vi "Teleop Cleaned by Oscar.vi"(10 "Match Info":T5={"Autonomous Elapsed Seconds"=0.0, "TeleOp Elapsed Seconds"=0.0, "Disabled Elapsed Seconds"=0.0, "Visited Autonomous"=FALSE, "Visited TeleOp"=FALSE, "Visited Disabled"=FALSE, "Autonomous Settings"={"Autonomous Style"=enum."Independent", "VI Refnum"=refnum}}, 11 "Call Context":T6) -> ()   [LabVIEW 2017]
doc: "This VI is called for each TeleOp packet received from the DS where the robot is not disabled. It is often used to read from the joysticks and update I/O or to update setpoints for timed control loops. It should complete and return within 20 milliseconds or it may miss DS packets."
uses:
  <vilib>/Rock Robotics/WPI/DriverStation/WPI_DriverStationDerivedRobotMode.ctl
  <vilib>/Rock Robotics/WPI/DriverStation/WPI_DriverStationMatch Info.ctl
  drive enum.ctl
  <vilib>/Rock Robotics/WPI/ThirdParty/Phoenix-LabVIEW/Motor Controller/Controls/CTRE_Phoenix_MotorControl_FeedbackDevice.ctl
  <vilib>/Rock Robotics/WPI/ThirdParty/Phoenix-LabVIEW/Motor Controller/Controls/CTRE_Phoenix_MotorControl_ControlMode.ctl
  <vilib>/Rock Robotics/WPI/Utilities/WPI_GetSetVariantRefNum.vi
  <vilib>/Rock Robotics/Network Tables/NT Write Boolean Array.vi
  <vilib>/Rock Robotics/Network Tables/NT Write Numeric Array.vi
  <vilib>/Rock Robotics/Network Tables/NT Read Boolean.vi
  <vilib>/Rock Robotics/Network Tables/NT Read Number.vi
  <vilib>/Rock Robotics/WPI/ThirdParty/Phoenix-LabVIEW/Motor Controller/Get/CTRE_Phoenix_MotorController_GetOutputCurrent_Enhanced.vi
  <vilib>/Rock Robotics/WPI/ThirdParty/Phoenix-LabVIEW/Motor Controller/Get/CTRE_Phoenix_MotorController_GetVoltage.vi
  <vilib>/Rock Robotics/WPI/ThirdParty/Phoenix-LabVIEW/Motor Controller/Get/CTRE_Phoenix_MotorController_GetClosedLoopData.vi
  <vilib>/Rock Robotics/WPI/ThirdParty/Phoenix-LabVIEW/Motor Controller/Get/CTRE_Phoenix_MotorController_GetSelectedSensorData.vi
panel:
  in  "X and Y values In":bool
  in  "Tab Control":T1(tab)
  in  "Cruise Velocity 3":i32=2000
  in  "Max Acceleration 3":i32=2000
  in  "Cruise Velocity 4":i32=2000
  in  "Max Acceleration 4":i32=2000
  in  "P 3":dbl format="%#_13g"
  in  "I 3":dbl format="%#_13g"
  in  "D 3":dbl format="%#_13g"
  in  "F 3":dbl=0.0095 format="%#_13g"
  in  "P 4":dbl format="%#_13g"
  in  "I 4":dbl format="%#_13g"
  in  "D 4":dbl format="%#_13g"
  in  "F 4":dbl=0.0095 format="%#_13g"
  out "Velocity (Raw Sensor Units per 100 ms) 6":i32
  out "Position (Raw Sensor Units) 6":i32
  out "Percent Output 4":dbl
  out "Velocity (Raw Sensor Units per 100 ms) 5":i32
  out "Position (Raw Sensor Units) 5":i32
  out "Percent Output 3":dbl
  out "Output Current 3":dbl
  out "Closed-loop Error 4":i32
  out "Output Current 4":dbl
  out "Closed-loop Error 3":i32
  in  "P":dbl format="%#_13g"
  in  "I":dbl format="%#_13g"
  in  "D":dbl format="%#_13g"
  in  "F":dbl=0.0095 format="%#_13g"
  in  "Cruise Velocity":i32=2000
  in  "Max Acceleration":i32=2000
  in  "Cruise Velocity 2":i32=2000
  in  "Max Acceleration 2":i32=2000
  in  "P 2":dbl format="%#_13g"
  in  "I 2":dbl format="%#_13g"
  in  "D 2":dbl format="%#_13g"
  in  "F 2":dbl=0.0095 format="%#_13g"
  out "Closed-loop Error 2":i32
  out "Percent Output 2":dbl
  out "Output Current 2":dbl
  out "Velocity (Raw Sensor Units per 100 ms) 4":i32
  out "Position (Raw Sensor Units) 4":i32
  out "Percent Output":dbl
  out "Output Current":dbl
  out "Velocity (Raw Sensor Units per 100 ms) 3":i32
  out "Position (Raw Sensor Units) 3":i32
  out "Closed-loop Error":i32
  out "Velocity (Raw Sensor Units per 100 ms) 7":i32
  out "Position (Raw Sensor Units) 7":i32
  out "Closed-loop Error 5":i32
  out "Percent Output 5":dbl
  out "Output Current 5":dbl
  out "Closed-loop Error 6":i32
  in  "Cruise Velocity 5":i32=2000
  in  "Max Acceleration 5":i32=2000
  in  "Cruise Velocity 6":i32=2000
  in  "Max Acceleration 6":i32=2000
  in  "P 5":dbl format="%#_13g"
  in  "D 5":dbl format="%#_13g"
  in  "F 5":dbl=0.0095 format="%#_13g"
  in  "I 5":dbl format="%#_13g"
  in  "P 6":dbl format="%#_13g"
  in  "I 6":dbl format="%#_13g"
  in  "D 6":dbl format="%#_13g"
  in  "F 6":dbl=0.0095 format="%#_13g"
  out "Velocity (Raw Sensor Units per 100 ms) 8":i32
  out "Position (Raw Sensor Units) 8":i32
  out "Percent Output 6":dbl
  out "Output Current 6":dbl
  out "Position (Raw Sensor Units)":i32
  out "Velocity (Raw Sensor Units per 100 ms)":i32
  out "Position (Raw Sensor Units) 2":i32
  out "Velocity (Raw Sensor Units per 100 ms) 2":i32
  in  "Y axis value":dbl
  in  "X axis value":dbl
  out "encoder position":i32(graph)
  out "X and Y":T2(graph)
  out "horizontal":dbl
  out "joystick output vertical":dbl
  out "closed loop error":T3(graph)
  out "voltage vs current left":T2(graph)
  out "voltage vs current right":T2(graph)
  out "Speed Closed Loop Plots":T4(graph)
  out "Sample Slider 0":dbl(slide) scale=0.0..5.0
  out "Sample Boolean 1":bool
  out "Sample Boolean 0":bool
  # "Joystick"
  # "Front Panel"
  # "what we want"
  # "actual"
  # "0.005740418607"
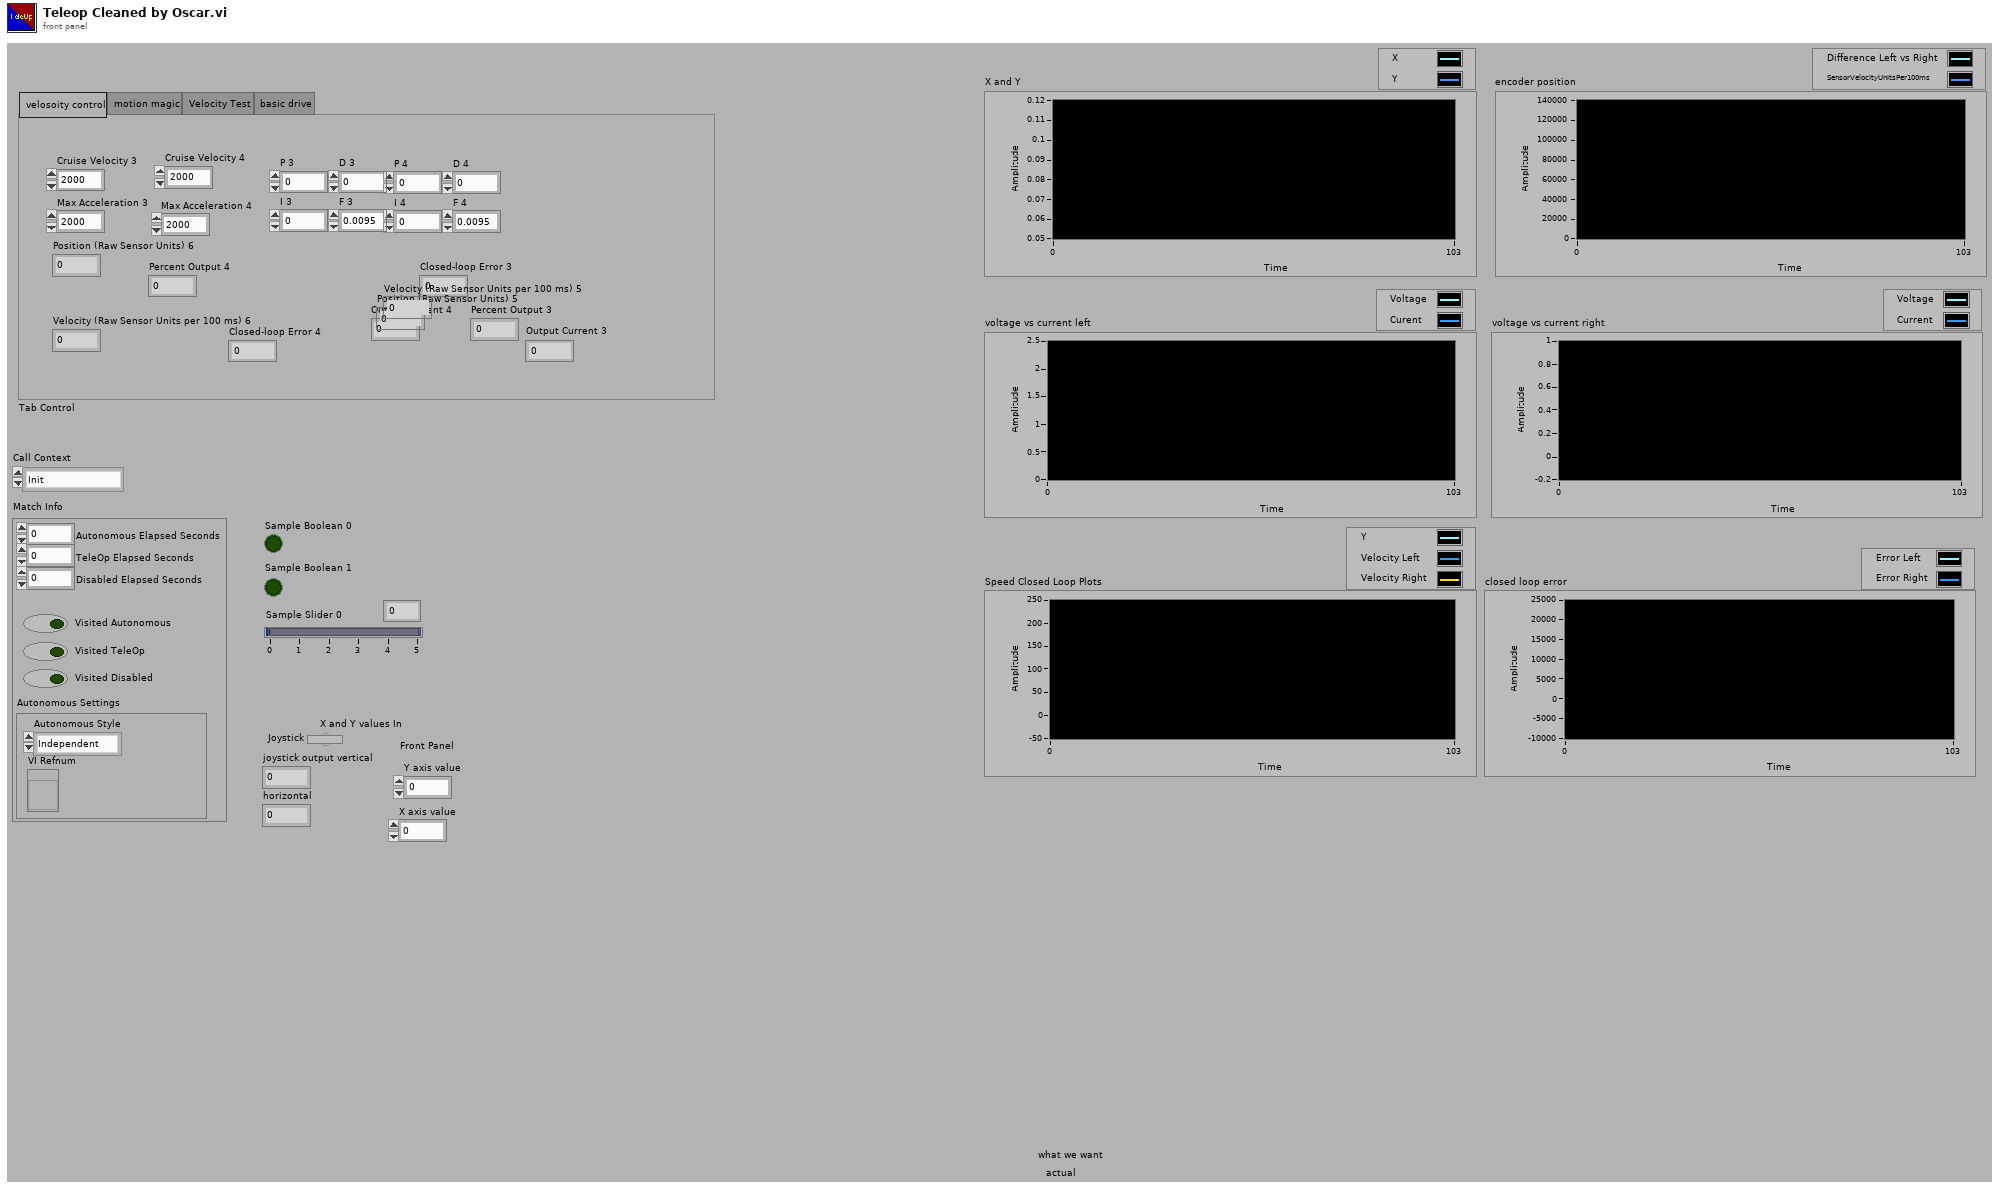
[diagram p1: front panel]
types:
  T1 = enum32{"velosoity control", "motion magic", "Velocity Test", "basic drive"}
  T2 = cluster{"Percent Output":dbl, "Output Current":dbl}
  T3 = cluster{"Closed-loop Error":i32, "Closed-loop Error":i32}
  T4 = cluster{dbl, "Velocity (Raw Sensor Units per 100 ms)":i32, "Velocity (Raw Sensor Units per 100 ms)":i32}
  T5 = typedef "WPI_DriverStationMatch Info.ctl" = cluster{"Autonomous Elapsed Seconds":dbl, "TeleOp Elapsed Seconds":dbl, "Disabled Elapsed Seconds":dbl, "Visited Autonomous":bool, "Visited TeleOp":bool, "Visited Disabled":bool, "Autonomous Settings":cluster{"Autonomous Style":enum16{"Iterative", "Independent"}, "VI Refnum":refnum<vi>}}
  T6 = typedef "WPI_DriverStationDerivedRobotMode.ctl" = enum16{"Init", "Execute", "Stop"}
  T7 = typedef "drive enum.ctl" = enum16{"velosoity control", "motion magic", "Velocity Test", "basic drive"}
  T8 = typedef "WPI_JoystickDevRef.ctl" = cluster{"Device":T9}
  T9 = typedef "WPI_JoystickDeviceEnum.ctl" = enum16{"USB 0", "USB 1", "USB 2", "USB 3", "USB 4", "USB 5"}
  T10 = typedef "WPI_RobotDriveDevRef.ctl" = cluster{"DevStatus":errorcluster, "Motors[]":T11[], "Square Inputs":bool, "Max Output":dbl}
  T11 = typedef "WPI_MotorControlDeviceRef.ctl" = cluster{"DeviceStatus":errorcluster, "Type":T12, "PWM":cluster{"PWM Channel":T13, "DeadBand":T14}, "CAN":cluster{"Device Number":u8, "SetOutput VI Ref":variant, "GetOutput VI Ref":variant, "Enable VI Ref":variant, "Disable VI Ref":variant, "Data":variant}, "Invert":bool, "DIO PWM":cluster{"PWM \"Enable\" Channel":T13, "DIOChannel":T15, "PWM Rate":dbl}}
  T12 = typedef "WPI_MotorControlType.ctl" = enum16{"PWM", "CAN", "DIO PWM"}
  T13 = typedef "FPGA_DIOPWMChannel.ctl" = enum8{"PWM 0", "PWM 1", "PWM 2", "PWM 3", "PWM 4", "PWM 5", "PWM 6", "PWM 7", "PWM 8", "PWM 9", "PWM MXP 0", "PWM MXP 1", "PWM MXP 2", "PWM MXP 3", "PWM MXP 4", "PWM MXP 5", "PWM MXP 6", "PWM MXP 7", "PWM MXP 8", "PWM MXP 9", "Invalid"}
  T14 = typedef "WPI_PWMDeadband.ctl" = cluster{"Name":string, "maxPositivePwm":i32, "minPositivePwm":i32, "centerPwm":i32, "maxNegativePwm":i32, "minNegativePwm":i32, "angularRange":u16}
  T15 = typedef "FPGA_DIOChannel.ctl" = enum8{"DIO 0", "DIO 1", "DIO 2", "DIO 3", "DIO 4", "DIO 5", "DIO 6", "DIO 7", "DIO 8", "DIO 9", "DIO MXP 0", "DIO MXP 1", "DIO MXP 2", "DIO MXP 3", "DIO MXP 4", "DIO MXP 5", "DIO MXP 6", "DIO MXP 7", "DIO MXP 8", "DIO MXP 9", "DIO MXP 10", "DIO MXP 11", "DIO MXP 12", "DIO MXP 13", "DIO MXP 14", "DIO MXP 15", "SPI Port CS1", "SPI Port CS2", "SPI Port CS3", "SPI Port MISO", "SPI Port MOSI", "Invalid"}
  T16 = typedef "CTRE_Phoenix_MotorControl_ControlMode.ctl" = u16
  T17 = typedef "CTRE_Phoenix_MotorControl_FeedbackDevice.ctl" = i8
  T18 = cluster{"Y axis value":dbl, "Velocity (Raw Sensor Units per 100 ms)":i32, "Velocity (Raw Sensor Units per 100 ms)":i32}
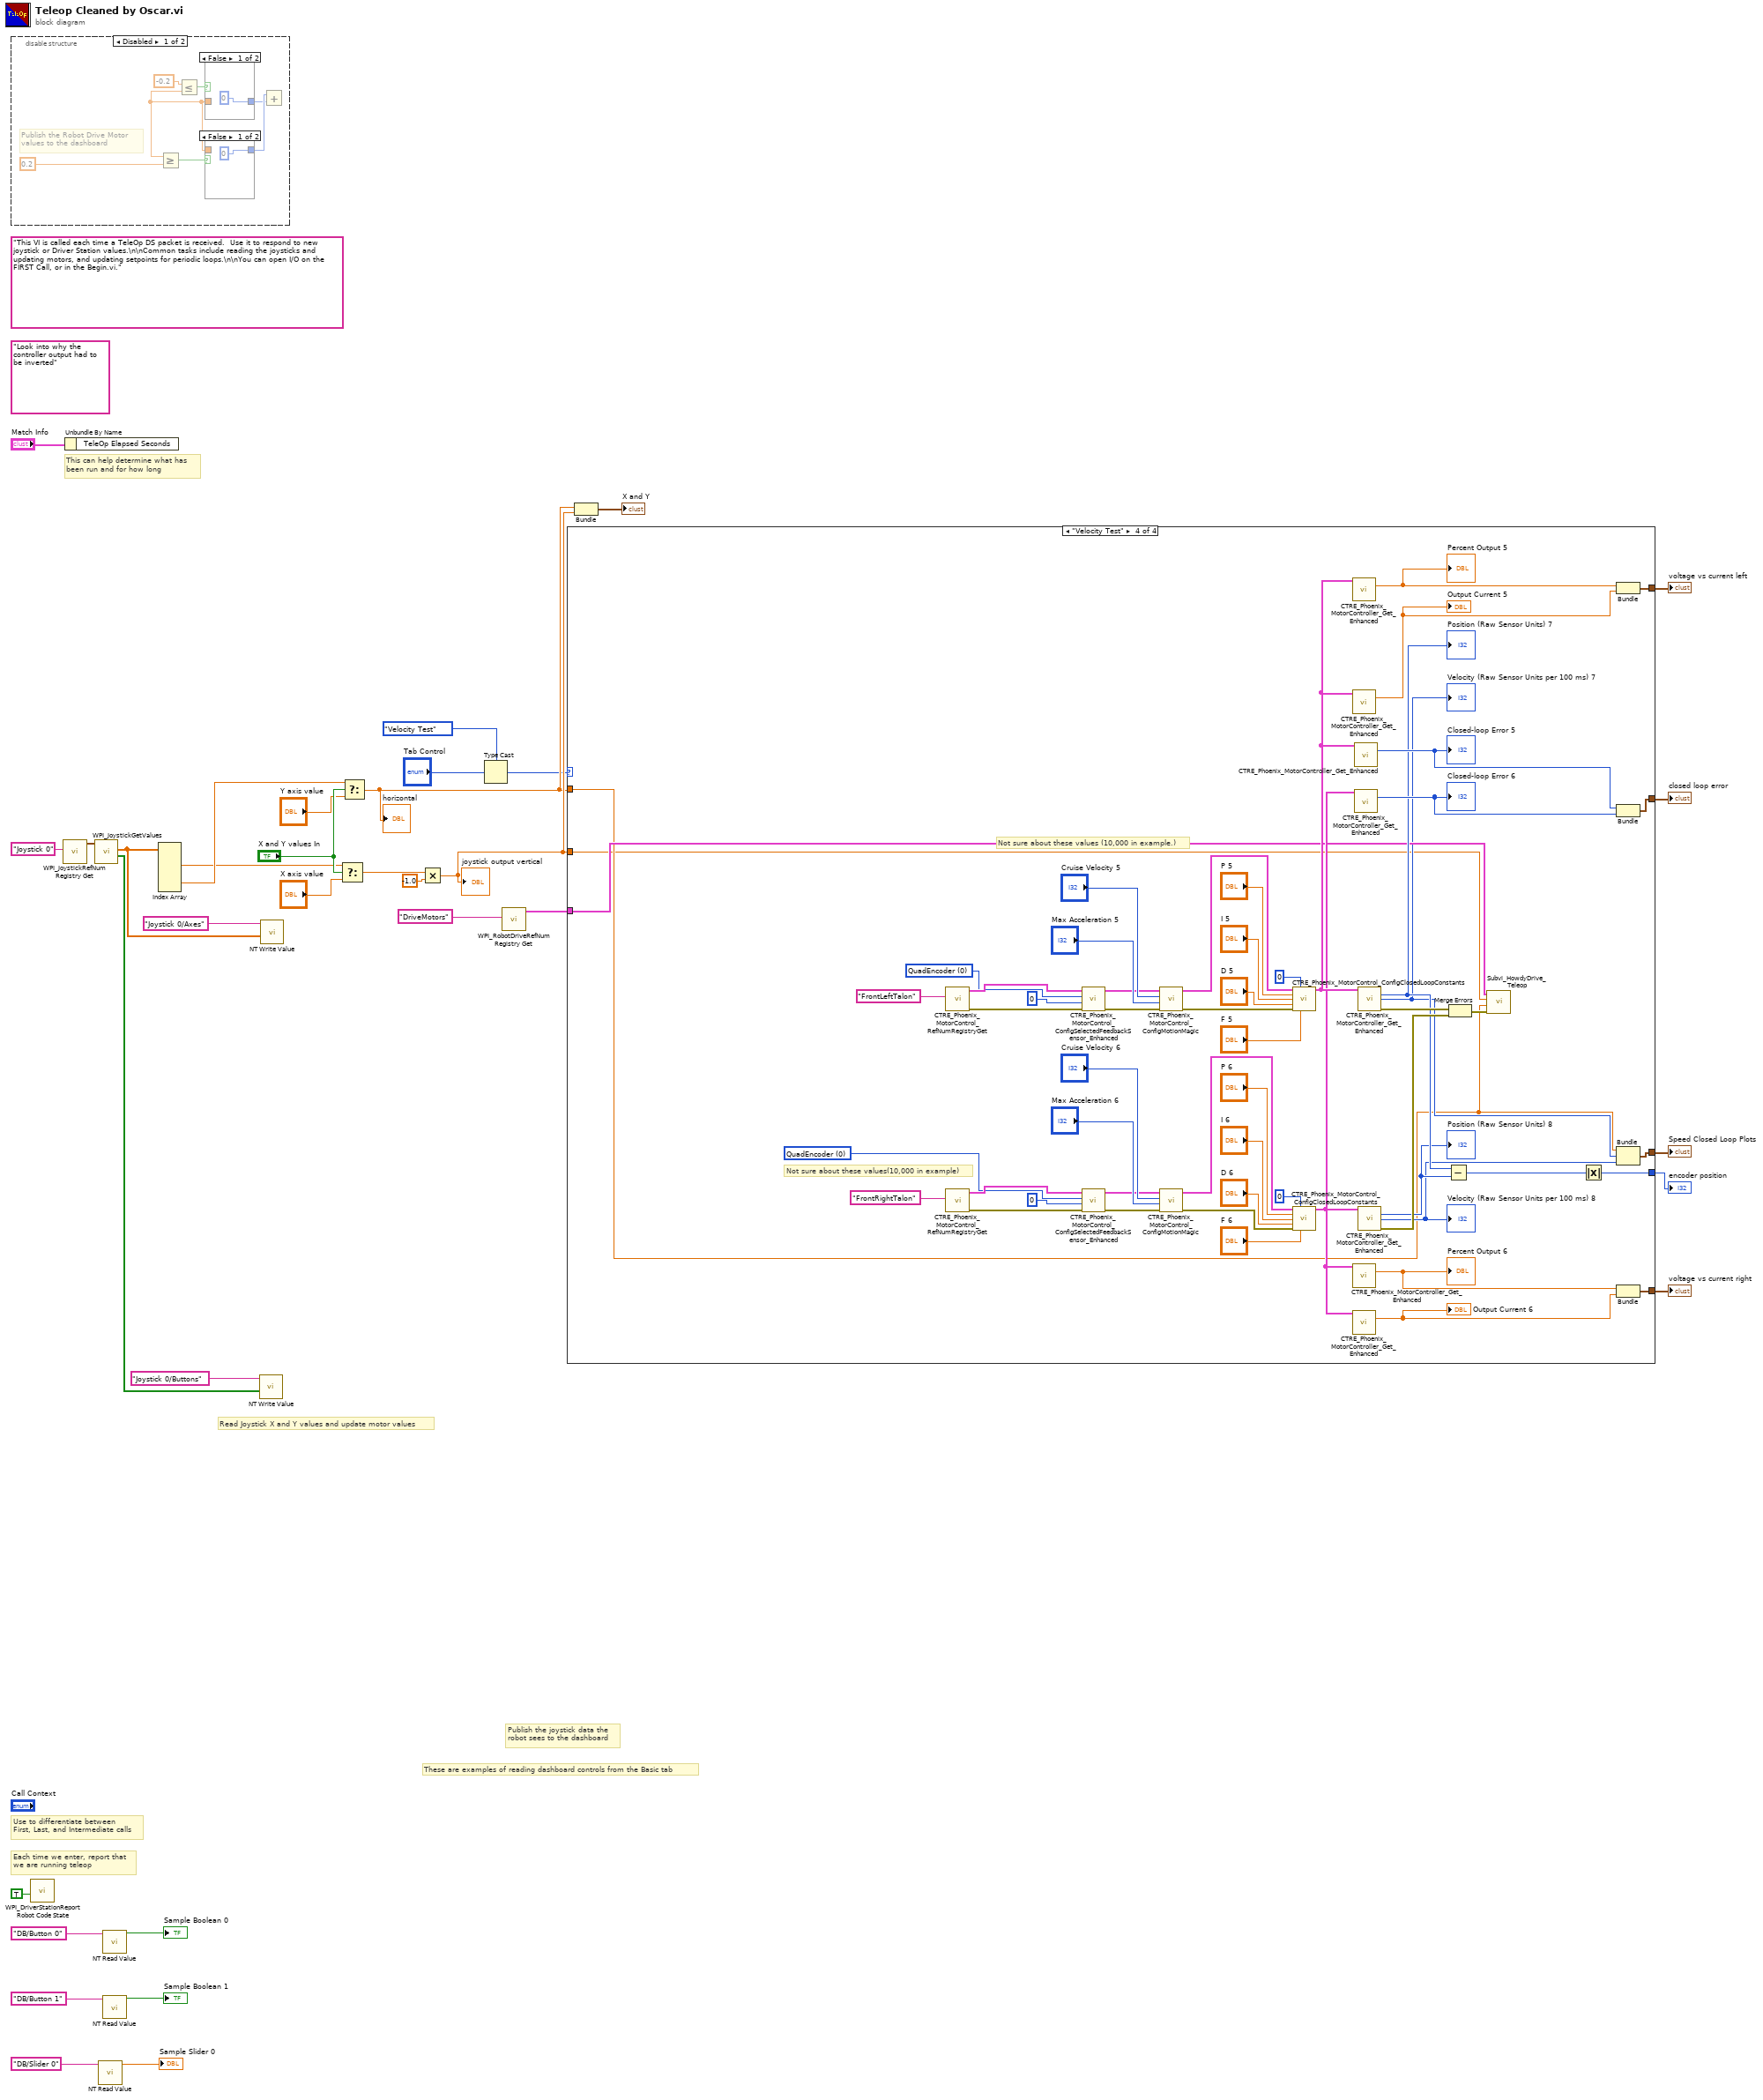
[diagram p0: block diagram]
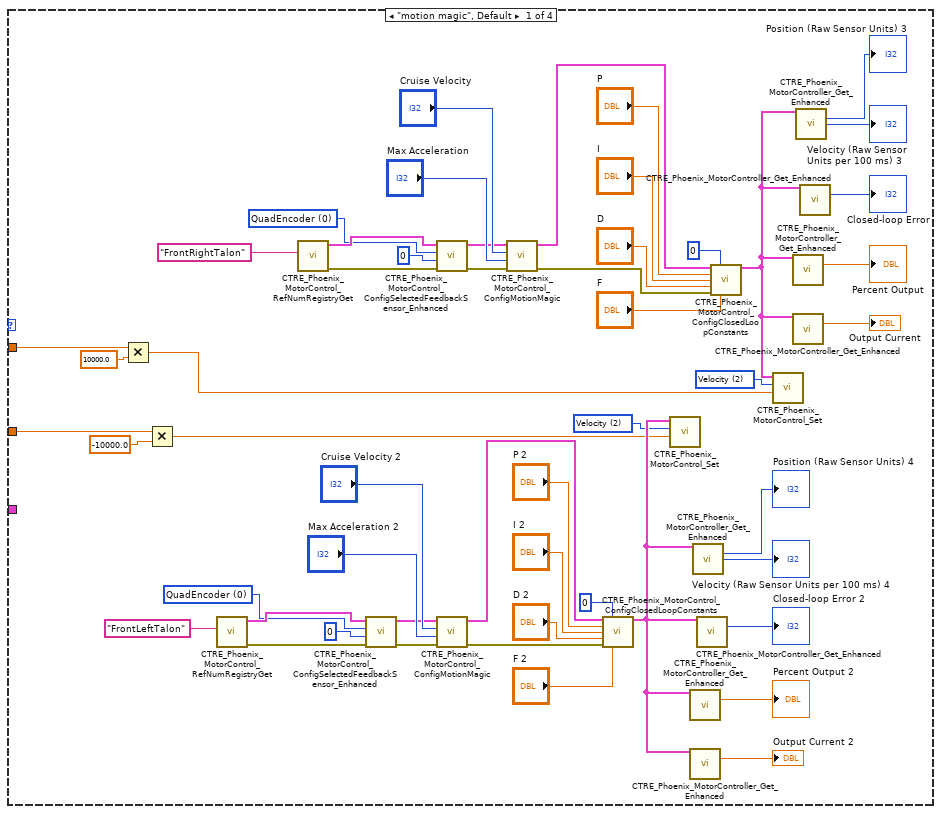
[diagram p5: hidden frame]
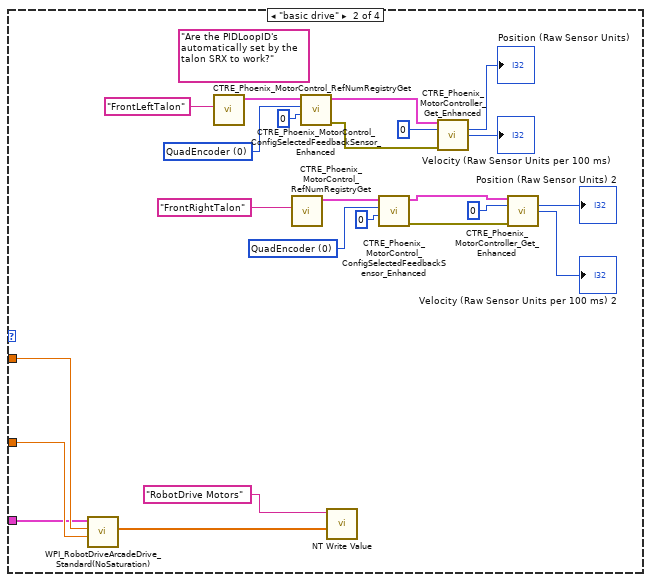
[diagram p6: hidden frame]
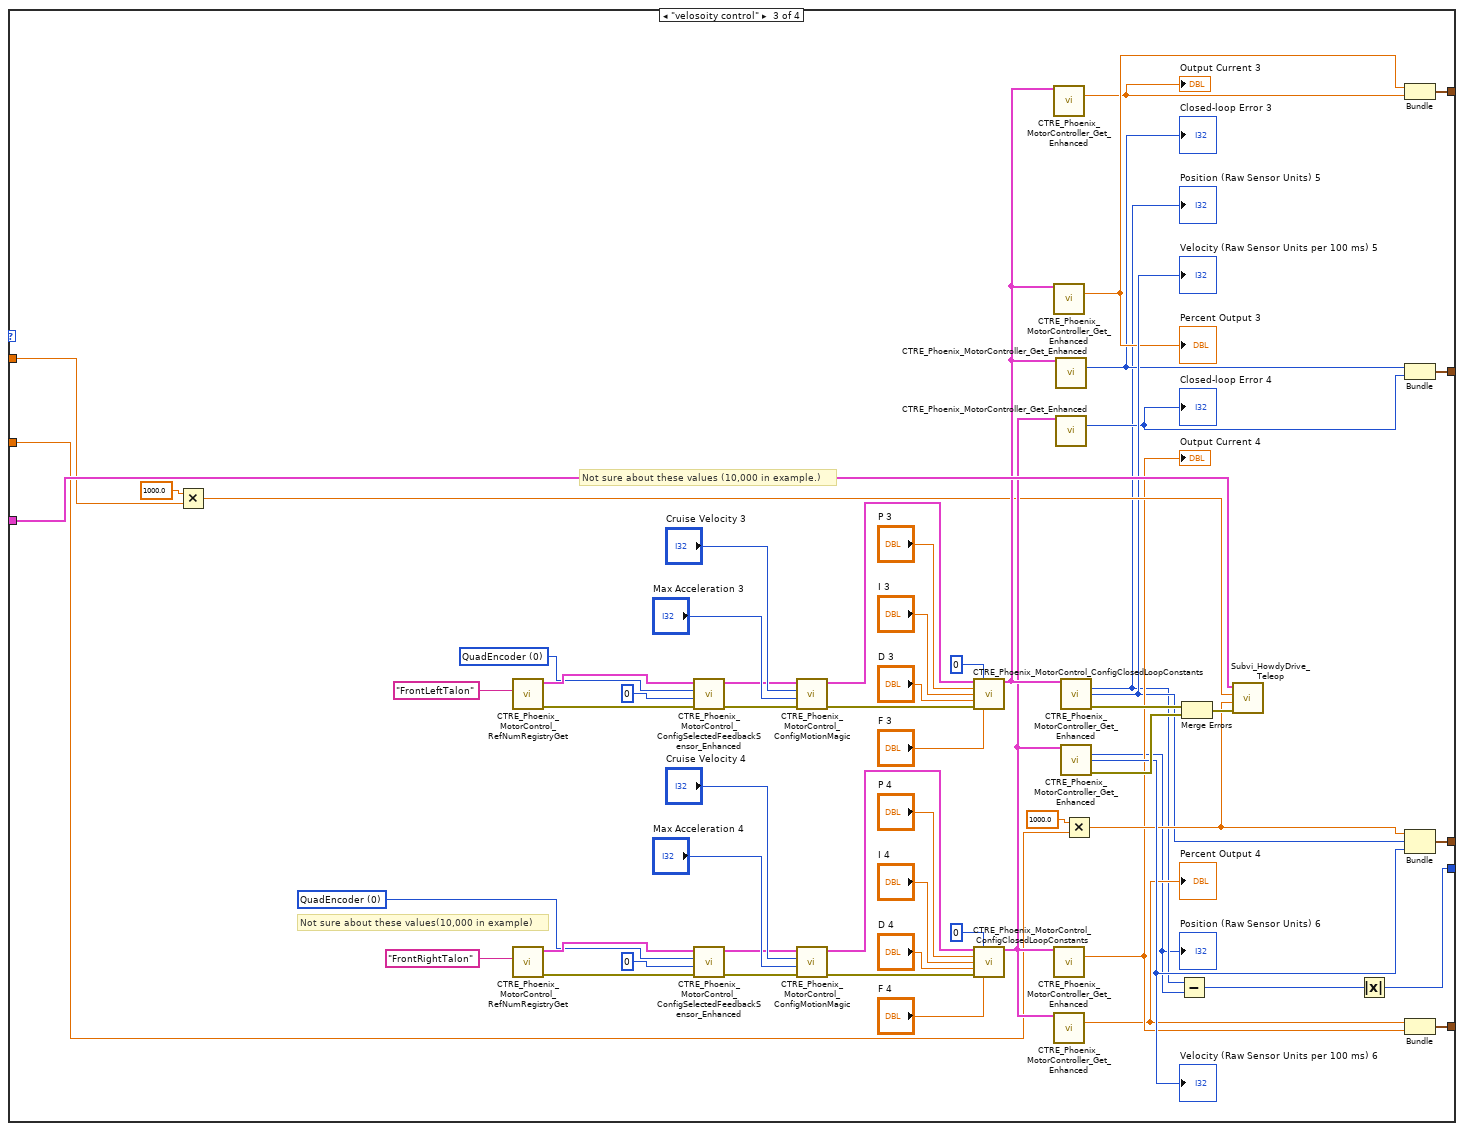
[diagram p7: hidden frame]
diagram:
  (unwired) "Look into why the controller output had to be inverted"
  (unwired) "This VI is called each time a TeleOp DS packet is received.  Use it to respond to new joystick or Driver Station values.\n\nCommon tasks include reading the joysticks and updating motors, and updating setpoints for periodic loops.\n\nYou can open I/O on the FIRST Call, or in the Begin.vi."
  # "These are examples of reading dashboard controls from the Basic tab"
  # "Publish the joystick data the\nrobot sees to the dashboard"
  # "Read Joystick X and Y values and update motor values"
  # "Each time we enter, report that\nwe are running teleop"
  # "Use to differentiate between\nFirst, Last, and Intermediate calls"
  # "This can help determine what has\nbeen run and for how long"
  n1 = disable-structure shown="Disabled" {
    frame Disabled {
      # "Publish the Robot Drive Motor\nvalues to the dashboard"
      n2 = Greater Or Equal?(y=0.2) -> (x=w37:dbl, x >= y?=w40:bool)
      n3 = Less Or Equal?(x=-0.2, y=w37) -> (x <= y?=w38:bool)
      n4 = case shown="False" w38 {
        tunnel: w37 -> [_ w43]
        tunnel: [0 w43] -> w35
        frame False {
        }
        frame True {
        }
      }
      n5 = case shown="False" w40 {
        tunnel: [0 w45] -> w36
        tunnel: w37 -> [_ w45]
        frame False {
        }
        frame True {
        }
      }
      n6 = Add(x=w36, y=w35) -> ()  [unwired: 1 out]
    }
    frame Enabled {
    }
  }
  n7 = call <vilib>:"WPI_DriverStationReport Robot Code State.vi"("TeleOp"=TRUE ("Autonomous")) -> ()  [unwired: 10 in, 1 out]
  n8 = call <vilib>:"WPI_JoystickRefNum Registry Get.vi"("refnum name"="Joystick 0") -> ("JoystickDevRef"=w30:T8)  [unwired: 1 in, 9 out]
  n9 = Unbundle By Name("Match Info") -> ()  [unwired: 1 out]
  n10 = call <vilib>:"WPI_JoystickGetValues.vi"("JoystickDevRef"=w30) -> ("Buttons"=w26:bool[], "Axes"=w27:dbl[])  [unwired: 6 in, 3 out]
  n11 = call-poly <vilib>:"NT Read Value.vi"("Name"="DB/Slider 0" ("refnum name")) -> ("Numeric"=→"Sample Slider 0":dbl)  [unwired: 9 in, 1 out]
  n12 = call-poly <vilib>:"NT Read Value.vi"("Name"="DB/Button 0" ("refnum name")) -> ("Boolean"=→"Sample Boolean 0":bool)  [unwired: 9 in, 1 out]
  n13 = call-poly <vilib>:"NT Read Value.vi"("Name"="DB/Button 1" ("refnum name")) -> ("Boolean"=→"Sample Boolean 1":bool)  [unwired: 9 in, 1 out]
  n14 = Index Array(array=w27) -> (element #2=w7:dbl, element #5=w8:dbl)  [unwired: 6 in, 4 out]
  n15 = call-poly <vilib>:"NT Write Value.vi"("Boolean Array"=w26, "Name"="Joystick 0/Buttons") -> ()  [unwired: 9 in, 1 out]
  n16 = call-poly <vilib>:"NT Write Value.vi"("Numeric Array"=w27, "Name"="Joystick 0/Axes") -> ()  [unwired: 9 in, 1 out]
  n17 = Select(t=w7, s="X and Y values In", f="X axis value") -> (s? t:f=w4:dbl)
  n18 = Select(t=w8, s="X and Y values In", f="Y axis value") -> (s? t:f=w5:dbl)
  "horizontal" <- w5
  n19 = Multiply(x=w4, y=-1.0) -> (x*y=w16:dbl)
  "joystick output vertical" <- w16
  n20 = Type Cast(type=drive_enum."Velocity Test", x="Tab Control") -> (*(type *) &x=w1:T7)
  n21 = call <vilib>:"WPI_RobotDriveRefNum Registry Get.vi"("refnum name"="DriveMotors") -> ("RobotDriveDevRef"=w18:T10)  [unwired: 1 in, 9 out]
  n22 = case shown="\"Velocity Test\"" w1 {
    tunnel: w16 -> [w48 w101 w139 w181]
    tunnel: w5 -> [w51 w100 w140 w182]
    tunnel: w18 -> [_ w99 w180 w190]
    tunnel: [_ _ w125 w189] -> w15
    tunnel: [_ _ w123 w187] -> w14
    tunnel: [_ _ w122 w185] -> w13
    tunnel: [_ _ w121 w186] -> w12
    tunnel: [_ _ w124 w188] -> w11
    frame "motion magic", Default {
      w56 = T16 2 items=["PercentOutput"=0, "Position"=1, "Velocity"=2, "Current"=3, "Follower"=5, "MotionProfile"=6, "MotionMagic"=7, "MotionMagicArc"=8, "MotionProfileArc"=10, "Disabled"=15] ("Control Mode")
      w53 = T17 0 items=["None"=-1, "QuadEncoder"=0, "Analog"=2, "Tachometer"=4, "Pulse Width Encoded Position"=8, "Sensor Sum (S0 + S1)"=9, "Sensor Difference (D0 - D1)"=10, "Remote Source 0"=11, "Remote Source 1"=12, "Software Emulated"=15] ("Feedback Device")
      w79 = T16 2 items=["PercentOutput"=0, "Position"=1, "Velocity"=2, "Current"=3, "Follower"=5, "MotionProfile"=6, "MotionMagic"=7, "MotionMagicArc"=8, "MotionProfileArc"=10, "Disabled"=15] ("Control Mode")
      w76 = T17 0 items=["None"=-1, "QuadEncoder"=0, "Analog"=2, "Tachometer"=4, "Pulse Width Encoded Position"=8, "Sensor Sum (S0 + S1)"=9, "Sensor Difference (D0 - D1)"=10, "Remote Source 0"=11, "Remote Source 1"=12, "Software Emulated"=15] ("Feedback Device")
      n23 = Multiply(x=w51, y=10000.0) -> (x*y=w46:dbl)
      n24 = Multiply(x=w48, y=-10000.0) -> (x*y=w47:dbl)
      n25 = call <vilib>:"CTRE_Phoenix_MotorControl_RefNumRegistryGet.vi"("refnum name"="FrontLeftTalon") -> ("error out"=w81:errorcluster, "PhoenixMotorControlDevRef"=w80:T11)  [unwired: 9 in]
      n26 = call <vilib>:"CTRE_Phoenix_MotorControl_RefNumRegistryGet.vi"("refnum name"="FrontRightTalon") -> ("error out"=w58:errorcluster, "PhoenixMotorControlDevRef"=w57:T11)  [unwired: 9 in]
      n27 = call <vilib>:"CTRE_Phoenix_MotorControl_ConfigSelectedFeedbackSensor_Enhanced.vi"("error in (no error)"=w81, "pidLoopIdx"=0, "Feedback Device"=w76, "PhoenixMotorControlDevRef"=w80) -> ("error out"=w83:errorcluster, "PhoenixMotorControlDevRef"=w82:T11)  [unwired: 6 in]
      n28 = call <vilib>:"CTRE_Phoenix_MotorControl_ConfigSelectedFeedbackSensor_Enhanced.vi"("error in (no error)"=w58, "pidLoopIdx"=0, "Feedback Device"=w53, "PhoenixMotorControlDevRef"=w57) -> ("error out"=w60:errorcluster, "PhoenixMotorControlDevRef"=w59:T11)  [unwired: 6 in]
      n29 = call <vilib>:"CTRE_Phoenix_MotorControl_ConfigMotionMagic.vi"("error in (no error)"=w83, "Acceleration"="Max Acceleration 2", "Cruise Velocity"="Cruise Velocity 2", "PhoenixMotorControlDevRef"=w82) -> ("error out"=w94:errorcluster, "PhoenixMotorControlDevRef"=w93:T11)  [unwired: 6 in]
      n30 = call <vilib>:"CTRE_Phoenix_MotorControl_ConfigMotionMagic.vi"("error in (no error)"=w60, "Acceleration"="Max Acceleration", "Cruise Velocity"="Cruise Velocity", "PhoenixMotorControlDevRef"=w59) -> ("error out"=w62:errorcluster, "PhoenixMotorControlDevRef"=w61:T11)  [unwired: 6 in]
      n31 = call <vilib>:"CTRE_Phoenix_MotorControl_ConfigClosedLoopConstants.vi"("PhoenixMotorControlDevRef"=w93, "slotIdx"=0, "P"="P 2", "I"="I 2", "D"="D 2", "error in (no error)"=w94, "F"="F 2") -> ("PhoenixMotorControlDevRef"=w97:T11)  [unwired: 7 in, 1 out]
      n32 = call <vilib>:"CTRE_Phoenix_MotorControl_Set.vi"("Output"=w47, "Control Mode"=w79, "PhoenixMotorControlDevRef"=w97) -> ()  [unwired: 7 in, 2 out]
      n33 = call-poly <vilib>:"CTRE_Phoenix_MotorController_Get_Enhanced.vi"("PhoenixMotorControlDevRef"=w97) -> ("Percent Output"=→"Percent Output 2":dbl)  [unwired: 10 in, 4 out]
      n34 = call-poly <vilib>:"CTRE_Phoenix_MotorController_Get_Enhanced.vi"("PhoenixMotorControlDevRef"=w97) -> ("Output Current"=→"Output Current 2":dbl)  [unwired: 12 in, 2 out]
      n35 = call-poly <vilib>:"CTRE_Phoenix_MotorController_Get_Enhanced.vi"("PhoenixMotorControlDevRef"=w97) -> ("Position (Raw Sensor Units)"=→"Position (Raw Sensor Units) 4":i32, "Velocity (Raw Sensor Units per 100 ms)"=→"Velocity (Raw Sensor Units per 100 ms) 4":i32)  [unwired: 11 in, 2 out]
      n36 = call-poly <vilib>:"CTRE_Phoenix_MotorController_Get_Enhanced.vi"("PhoenixMotorControlDevRef"=w97) -> ("Closed-loop Error"=→"Closed-loop Error 2":i32)  [unwired: 9 in, 5 out]
      n37 = call <vilib>:"CTRE_Phoenix_MotorControl_ConfigClosedLoopConstants.vi"("PhoenixMotorControlDevRef"=w61, "slotIdx"=0, "P"="P", "I"="I", "D"="D", "error in (no error)"=w62, "F"="F") -> ("PhoenixMotorControlDevRef"=w74:T11)  [unwired: 7 in, 1 out]
      n38 = call <vilib>:"CTRE_Phoenix_MotorControl_Set.vi"("Output"=w46, "Control Mode"=w56, "PhoenixMotorControlDevRef"=w74) -> ()  [unwired: 7 in, 2 out]
      n39 = call-poly <vilib>:"CTRE_Phoenix_MotorController_Get_Enhanced.vi"("PhoenixMotorControlDevRef"=w74) -> ("Percent Output"=→"Percent Output":dbl)  [unwired: 10 in, 4 out]
      n40 = call-poly <vilib>:"CTRE_Phoenix_MotorController_Get_Enhanced.vi"("PhoenixMotorControlDevRef"=w74) -> ("Output Current"=→"Output Current":dbl)  [unwired: 12 in, 2 out]
      n41 = call-poly <vilib>:"CTRE_Phoenix_MotorController_Get_Enhanced.vi"("PhoenixMotorControlDevRef"=w74) -> ("Position (Raw Sensor Units)"=→"Position (Raw Sensor Units) 3":i32, "Velocity (Raw Sensor Units per 100 ms)"=→"Velocity (Raw Sensor Units per 100 ms) 3":i32)  [unwired: 11 in, 2 out]
      n42 = call-poly <vilib>:"CTRE_Phoenix_MotorController_Get_Enhanced.vi"("PhoenixMotorControlDevRef"=w74) -> ("Closed-loop Error"=→"Closed-loop Error":i32)  [unwired: 9 in, 5 out]
    }
    frame "basic drive" {
      (unwired) "Are the PIDLoopID's automatically set by the talon SRX to work?"
      w113 = T17 0 items=["None"=-1, "QuadEncoder"=0, "Analog"=2, "Tachometer"=4, "Pulse Width Encoded Position"=8, "Sensor Sum (S0 + S1)"=9, "Sensor Difference (D0 - D1)"=10, "Remote Source 0"=11, "Remote Source 1"=12, "Software Emulated"=15] ("Feedback Device")
      w120 = T17 0 items=["None"=-1, "QuadEncoder"=0, "Analog"=2, "Tachometer"=4, "Pulse Width Encoded Position"=8, "Sensor Sum (S0 + S1)"=9, "Sensor Difference (D0 - D1)"=10, "Remote Source 0"=11, "Remote Source 1"=12, "Software Emulated"=15] ("Feedback Device")
      n43 = call <vilib>:"WPI_RobotDriveArcadeDrive_Standard(NoSaturation).vi"("Y axis value"=w101, "X axis value"=w100, "RobotDriveDevRef"=w99) -> ("Motor Values"=w102:dbl[])  [unwired: 1 in, 7 out]
      n44 = call <vilib>:"CTRE_Phoenix_MotorControl_RefNumRegistryGet.vi"("refnum name"="FrontLeftTalon") -> ("PhoenixMotorControlDevRef"=w114:T11)  [unwired: 9 in, 1 out]
      n45 = call <vilib>:"CTRE_Phoenix_MotorControl_RefNumRegistryGet.vi"("refnum name"="FrontRightTalon") -> ("PhoenixMotorControlDevRef"=w106:T11)  [unwired: 9 in, 1 out]
      n46 = call <vilib>:"CTRE_Phoenix_MotorControl_ConfigSelectedFeedbackSensor_Enhanced.vi"("pidLoopIdx"=0, "Feedback Device"=w120, "PhoenixMotorControlDevRef"=w114) -> ("error out"=w118:errorcluster, "PhoenixMotorControlDevRef"=w119:T11)  [unwired: 7 in]
      n47 = call-poly <vilib>:"NT Write Value.vi"("Numeric Array"=w102, "Name"="RobotDrive Motors") -> ()  [unwired: 9 in, 1 out]
      n48 = call <vilib>:"CTRE_Phoenix_MotorControl_ConfigSelectedFeedbackSensor_Enhanced.vi"("pidLoopIdx"=0, "Feedback Device"=w113, "PhoenixMotorControlDevRef"=w106) -> ("error out"=w111:errorcluster, "PhoenixMotorControlDevRef"=w112:T11)  [unwired: 7 in]
      n49 = call-poly <vilib>:"CTRE_Phoenix_MotorController_Get_Enhanced.vi"("PhoenixMotorControlDevRef"=w119, "pidLoopIdx"=u32 0, "error in"=w118) -> ("Position (Raw Sensor Units)"=→"Position (Raw Sensor Units)":i32, "Velocity (Raw Sensor Units per 100 ms)"=→"Velocity (Raw Sensor Units per 100 ms)":i32)  [unwired: 9 in, 2 out]
      n50 = call-poly <vilib>:"CTRE_Phoenix_MotorController_Get_Enhanced.vi"("PhoenixMotorControlDevRef"=w112, "pidLoopIdx"=u32 0, "error in"=w111) -> ("Position (Raw Sensor Units)"=→"Position (Raw Sensor Units) 2":i32, "Velocity (Raw Sensor Units per 100 ms)"=→"Velocity (Raw Sensor Units per 100 ms) 2":i32)  [unwired: 9 in, 2 out]
    }
    frame "velosoity control" {
      w147 = T17 0 items=["None"=-1, "QuadEncoder"=0, "Analog"=2, "Tachometer"=4, "Pulse Width Encoded Position"=8, "Sensor Sum (S0 + S1)"=9, "Sensor Difference (D0 - D1)"=10, "Remote Source 0"=11, "Remote Source 1"=12, "Software Emulated"=15] ("Feedback Device")
      w164 = T17 0 items=["None"=-1, "QuadEncoder"=0, "Analog"=2, "Tachometer"=4, "Pulse Width Encoded Position"=8, "Sensor Sum (S0 + S1)"=9, "Sensor Difference (D0 - D1)"=10, "Remote Source 0"=11, "Remote Source 1"=12, "Software Emulated"=15] ("Feedback Device")
      # "Not sure about these values (10,000 in example.)"
      # "Not sure about these values(10,000 in example)"
      n51 = Multiply(x=1000.0, y=w140) -> (x*y=w138:dbl)
      n52 = call <vilib>:"CTRE_Phoenix_MotorControl_RefNumRegistryGet.vi"("refnum name"="FrontLeftTalon") -> ("error out"=w168:errorcluster, "PhoenixMotorControlDevRef"=w167:T11)  [unwired: 9 in]
      n53 = call <vilib>:"CTRE_Phoenix_MotorControl_RefNumRegistryGet.vi"("refnum name"="FrontRightTalon") -> ("error out"=w151:errorcluster, "PhoenixMotorControlDevRef"=w150:T11)  [unwired: 9 in]
      n54 = call <vilib>:"CTRE_Phoenix_MotorControl_ConfigSelectedFeedbackSensor_Enhanced.vi"("error in (no error)"=w168, "pidLoopIdx"=0, "Feedback Device"=w164, "PhoenixMotorControlDevRef"=w167) -> ("error out"=w170:errorcluster, "PhoenixMotorControlDevRef"=w169:T11)  [unwired: 6 in]
      n55 = call <vilib>:"CTRE_Phoenix_MotorControl_ConfigSelectedFeedbackSensor_Enhanced.vi"("error in (no error)"=w151, "pidLoopIdx"=0, "Feedback Device"=w147, "PhoenixMotorControlDevRef"=w150) -> ("error out"=w153:errorcluster, "PhoenixMotorControlDevRef"=w152:T11)  [unwired: 6 in]
      n56 = call <vilib>:"CTRE_Phoenix_MotorControl_ConfigMotionMagic.vi"("error in (no error)"=w170, "Acceleration"="Max Acceleration 3", "Cruise Velocity"="Cruise Velocity 3", "PhoenixMotorControlDevRef"=w169) -> ("error out"=w176:errorcluster, "PhoenixMotorControlDevRef"=w175:T11)  [unwired: 6 in]
      n57 = call <vilib>:"CTRE_Phoenix_MotorControl_ConfigMotionMagic.vi"("error in (no error)"=w153, "Acceleration"="Max Acceleration 4", "Cruise Velocity"="Cruise Velocity 4", "PhoenixMotorControlDevRef"=w152) -> ("error out"=w155:errorcluster, "PhoenixMotorControlDevRef"=w154:T11)  [unwired: 6 in]
      n58 = call <vilib>:"CTRE_Phoenix_MotorControl_ConfigClosedLoopConstants.vi"("PhoenixMotorControlDevRef"=w175, "slotIdx"=0, "P"="P 3", "I"="I 3", "D"="D 3", "error in (no error)"=w176, "F"="F 3") -> ("PhoenixMotorControlDevRef"=w179:T11)  [unwired: 7 in, 1 out]
      n59 = call <vilib>:"CTRE_Phoenix_MotorControl_ConfigClosedLoopConstants.vi"("PhoenixMotorControlDevRef"=w154, "slotIdx"=0, "P"="P 4", "I"="I 4", "D"="D 4", "error in (no error)"=w155, "F"="F 4") -> ("PhoenixMotorControlDevRef"=w162:T11)  [unwired: 7 in, 1 out]
      n60 = call-poly <vilib>:"CTRE_Phoenix_MotorController_Get_Enhanced.vi"("PhoenixMotorControlDevRef"=w179) -> ("Output Current"=w131:dbl)  [unwired: 12 in, 2 out]
      "Output Current 3" <- w131
      n61 = call-poly <vilib>:"CTRE_Phoenix_MotorController_Get_Enhanced.vi"("PhoenixMotorControlDevRef"=w179) -> ("Percent Output"=w132:dbl)  [unwired: 10 in, 4 out]
      "Percent Output 3" <- w132
      n62 = call-poly <vilib>:"CTRE_Phoenix_MotorController_Get_Enhanced.vi"("PhoenixMotorControlDevRef"=w162) -> ("Output Current"=w135:dbl)  [unwired: 12 in, 2 out]
      "Output Current 4" <- w135
      n63 = call-poly <vilib>:"CTRE_Phoenix_MotorController_Get_Enhanced.vi"("PhoenixMotorControlDevRef"=w162) -> ("Percent Output"=w134:dbl)  [unwired: 10 in, 4 out]
      "Percent Output 4" <- w134
      n64 = call-poly <vilib>:"CTRE_Phoenix_MotorController_Get_Enhanced.vi"("PhoenixMotorControlDevRef"=w179) -> ("Closed-loop Error"=w130:i32)  [unwired: 9 in, 5 out]
      "Closed-loop Error 3" <- w130
      n65 = call-poly <vilib>:"CTRE_Phoenix_MotorController_Get_Enhanced.vi"("PhoenixMotorControlDevRef"=w162) -> ("Closed-loop Error"=w129:i32)  [unwired: 9 in, 5 out]
      "Closed-loop Error 4" <- w129
      n66 = call-poly <vilib>:"CTRE_Phoenix_MotorController_Get_Enhanced.vi"("PhoenixMotorControlDevRef"=w179) -> ("Position (Raw Sensor Units)"=w128:i32, "Velocity (Raw Sensor Units per 100 ms)"=w133:i32, "error out"=w144:errorcluster)  [unwired: 11 in, 1 out]
      "Velocity (Raw Sensor Units per 100 ms) 5" <- w133
      "Position (Raw Sensor Units) 5" <- w128
      n67 = call-poly <vilib>:"CTRE_Phoenix_MotorController_Get_Enhanced.vi"("PhoenixMotorControlDevRef"=w162) -> ("Position (Raw Sensor Units)"=w127:i32, "Velocity (Raw Sensor Units per 100 ms)"=w137:i32, "error out"=w145:errorcluster)  [unwired: 11 in, 1 out]
      "Velocity (Raw Sensor Units per 100 ms) 6" <- w137
      "Position (Raw Sensor Units) 6" <- w127
      n68 = Multiply(x=1000.0, y=w139) -> (x*y=w136:dbl)
      n69 = Subtract(x=w128, y=w127) -> (x-y=w126:i32)
      n70 = Merge Errors(w144, w145) -> (w143:errorcluster)
      n71 = call "Subvi_HowdyDrive_Teleop.vi"("error in (no error)"=w143, "Y axis value"=w136, "X axis value"=w138, "RobotDriveDevRef"=w180) -> ()  [unwired: 6 in, 2 out]
      n72 = Absolute Value(x=w126) -> (abs(x)=w125:i32)
      n73 = Bundle("Percent Output"=w132, "Output Current"=w131) -> (w123:T2)  [unwired: 1 in]
      n74 = Bundle("Closed-loop Error"=w130, "Closed-loop Error"=w129) -> (w124:T3)  [unwired: 1 in]
      n75 = Bundle(w136, "Velocity (Raw Sensor Units per 100 ms)"=w133, "Velocity (Raw Sensor Units per 100 ms)"=w137) -> (w122:T4)  [unwired: 1 in]
      n76 = Bundle("Percent Output"=w134, "Output Current"=w135) -> (w121:T2)  [unwired: 1 in]
    }
    frame "Velocity Test" {
      w204 = T17 0 items=["None"=-1, "QuadEncoder"=0, "Analog"=2, "Tachometer"=4, "Pulse Width Encoded Position"=8, "Sensor Sum (S0 + S1)"=9, "Sensor Difference (D0 - D1)"=10, "Remote Source 0"=11, "Remote Source 1"=12, "Software Emulated"=15] ("Feedback Device")
      w221 = T17 0 items=["None"=-1, "QuadEncoder"=0, "Analog"=2, "Tachometer"=4, "Pulse Width Encoded Position"=8, "Sensor Sum (S0 + S1)"=9, "Sensor Difference (D0 - D1)"=10, "Remote Source 0"=11, "Remote Source 1"=12, "Software Emulated"=15] ("Feedback Device")
      # "Not sure about these values (10,000 in example.)"
      # "Not sure about these values(10,000 in example)"
      n77 = call <vilib>:"CTRE_Phoenix_MotorControl_RefNumRegistryGet.vi"("refnum name"="FrontLeftTalon") -> ("error out"=w225:errorcluster, "PhoenixMotorControlDevRef"=w224:T11)  [unwired: 9 in]
      n78 = call <vilib>:"CTRE_Phoenix_MotorControl_RefNumRegistryGet.vi"("refnum name"="FrontRightTalon") -> ("error out"=w208:errorcluster, "PhoenixMotorControlDevRef"=w207:T11)  [unwired: 9 in]
      n79 = call <vilib>:"CTRE_Phoenix_MotorControl_ConfigSelectedFeedbackSensor_Enhanced.vi"("error in (no error)"=w225, "pidLoopIdx"=0, "Feedback Device"=w221, "PhoenixMotorControlDevRef"=w224) -> ("error out"=w227:errorcluster, "PhoenixMotorControlDevRef"=w226:T11)  [unwired: 6 in]
      n80 = call <vilib>:"CTRE_Phoenix_MotorControl_ConfigSelectedFeedbackSensor_Enhanced.vi"("error in (no error)"=w208, "pidLoopIdx"=0, "Feedback Device"=w204, "PhoenixMotorControlDevRef"=w207) -> ("error out"=w210:errorcluster, "PhoenixMotorControlDevRef"=w209:T11)  [unwired: 6 in]
      n81 = call <vilib>:"CTRE_Phoenix_MotorControl_ConfigMotionMagic.vi"("error in (no error)"=w227, "Acceleration"="Max Acceleration 5", "Cruise Velocity"="Cruise Velocity 5", "PhoenixMotorControlDevRef"=w226) -> ("error out"=w233:errorcluster, "PhoenixMotorControlDevRef"=w232:T11)  [unwired: 6 in]
      n82 = call <vilib>:"CTRE_Phoenix_MotorControl_ConfigMotionMagic.vi"("error in (no error)"=w210, "Acceleration"="Max Acceleration 6", "Cruise Velocity"="Cruise Velocity 6", "PhoenixMotorControlDevRef"=w209) -> ("error out"=w212:errorcluster, "PhoenixMotorControlDevRef"=w211:T11)  [unwired: 6 in]
      n83 = call <vilib>:"CTRE_Phoenix_MotorControl_ConfigClosedLoopConstants.vi"("PhoenixMotorControlDevRef"=w232, "slotIdx"=0, "P"="P 5", "I"="I 5", "D"="D 5", "error in (no error)"=w233, "F"="F 5") -> ("PhoenixMotorControlDevRef"=w236:T11)  [unwired: 7 in, 1 out]
      n84 = call <vilib>:"CTRE_Phoenix_MotorControl_ConfigClosedLoopConstants.vi"("PhoenixMotorControlDevRef"=w211, "slotIdx"=0, "P"="P 6", "I"="I 6", "D"="D 6", "error in (no error)"=w212, "F"="F 6") -> ("PhoenixMotorControlDevRef"=w219:T11)  [unwired: 7 in, 1 out]
      n85 = call-poly <vilib>:"CTRE_Phoenix_MotorController_Get_Enhanced.vi"("PhoenixMotorControlDevRef"=w236) -> ("Percent Output"=w197:dbl)  [unwired: 10 in, 4 out]
      "Percent Output 5" <- w197
      n86 = call-poly <vilib>:"CTRE_Phoenix_MotorController_Get_Enhanced.vi"("PhoenixMotorControlDevRef"=w236) -> ("Output Current"=w196:dbl)  [unwired: 12 in, 2 out]
      "Output Current 5" <- w196
      n87 = call-poly <vilib>:"CTRE_Phoenix_MotorController_Get_Enhanced.vi"("PhoenixMotorControlDevRef"=w219) -> ("Percent Output"=w198:dbl)  [unwired: 10 in, 4 out]
      "Percent Output 6" <- w198
      n88 = call-poly <vilib>:"CTRE_Phoenix_MotorController_Get_Enhanced.vi"("PhoenixMotorControlDevRef"=w219) -> ("Output Current"=w199:dbl)  [unwired: 12 in, 2 out]
      "Output Current 6" <- w199
      n89 = call-poly <vilib>:"CTRE_Phoenix_MotorController_Get_Enhanced.vi"("PhoenixMotorControlDevRef"=w236) -> ("Closed-loop Error"=w195:i32)  [unwired: 9 in, 5 out]
      "Closed-loop Error 5" <- w195
      n90 = call-poly <vilib>:"CTRE_Phoenix_MotorController_Get_Enhanced.vi"("PhoenixMotorControlDevRef"=w219) -> ("Closed-loop Error"=w194:i32)  [unwired: 9 in, 5 out]
      "Closed-loop Error 6" <- w194
      n91 = call-poly <vilib>:"CTRE_Phoenix_MotorController_Get_Enhanced.vi"("PhoenixMotorControlDevRef"=w236) -> ("Position (Raw Sensor Units)"=w193:i32, "Velocity (Raw Sensor Units per 100 ms)"=w184:i32, "error out"=w201:errorcluster)  [unwired: 11 in, 1 out]
      "Velocity (Raw Sensor Units per 100 ms) 7" <- w184
      "Position (Raw Sensor Units) 7" <- w193
      n92 = call-poly <vilib>:"CTRE_Phoenix_MotorController_Get_Enhanced.vi"("PhoenixMotorControlDevRef"=w219) -> ("Position (Raw Sensor Units)"=w192:i32, "Velocity (Raw Sensor Units per 100 ms)"=w183:i32, "error out"=w202:errorcluster)  [unwired: 11 in, 1 out]
      "Velocity (Raw Sensor Units per 100 ms) 8" <- w183
      "Position (Raw Sensor Units) 8" <- w192
      n93 = Subtract(x=w193, y=w192) -> (x-y=w191:i32)
      n94 = Merge Errors(w201, w202) -> (w200:errorcluster)
      n95 = call "Subvi_HowdyDrive_Teleop.vi"("error in (no error)"=w200, "Y axis value"=w182, "X axis value"=w181, "RobotDriveDevRef"=w190) -> ()  [unwired: 6 in, 2 out]
      n96 = Absolute Value(x=w191) -> (abs(x)=w189:i32)
      n97 = Bundle("Percent Output"=w197, "Output Current"=w196) -> (w187:T2)  [unwired: 1 in]
      n98 = Bundle("Closed-loop Error"=w195, "Closed-loop Error"=w194) -> (w188:T3)  [unwired: 1 in]
      n99 = Bundle("Y axis value"=w182, "Velocity (Raw Sensor Units per 100 ms)"=w184, "Velocity (Raw Sensor Units per 100 ms)"=w183) -> (w185:T18)  [unwired: 1 in]
      n100 = Bundle("Percent Output"=w198, "Output Current"=w199) -> (w186:T2)  [unwired: 1 in]
    }
  }
  "encoder position" <- w15
  "closed loop error" <- w11
  "voltage vs current left" <- w14
  "Speed Closed Loop Plots" <- w13
  "voltage vs current right" <- w12
  n101 = Bundle("Y axis value"=w5, w16) -> (→"X and Y":cluster{"Y axis value":dbl, dbl})  [unwired: 1 in]
